vi "Config path --constant.vi"() -> (3 "appended path":path)   [LabVIEW 2020]
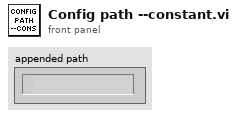
[diagram p1: front panel]
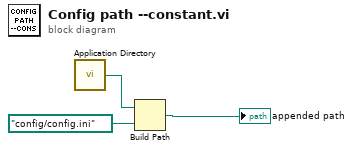
[diagram p0: block diagram]
diagram:
  n1 = call <vilib>:"Application Directory.vi"() -> ("Application Directory"=w1:path)
  n2 = Build Path(base path=w1, name or relative path=path "config/config.ini" ("configuration file path")) -> (appended path=→"appended path":path)
